vi "OnChunk.vi"(8 "Error In":errorcluster, 11 "JSON Tree In":variant) -> (0 "Error Out":errorcluster, 1 "Payload":variant, 2 "SessionId":string, 3 "JSON Tree Out":variant)   [LabVIEW 2017, in "LiteAgentSDK.lvlib"]
uses:
  LiteAgentSDK.lvlib
  <vilib>/LVH/i3 JSON/JSON Parsing/Get Object Parameter Files/Get Object Parameter - String.vi
  <vilib>/LVH/i3 JSON/JSON Parsing/Get Object Parameter Files/Get Object Parameter - Object.vi
  <vilib>/LVH/i3 JSON/i3-json.lvlib
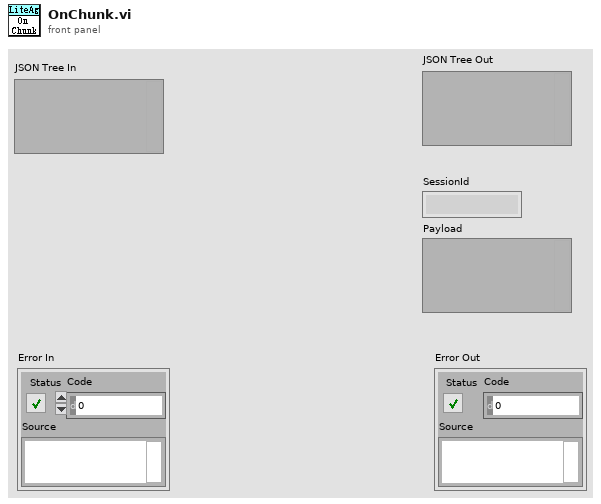
[diagram p1: front panel]
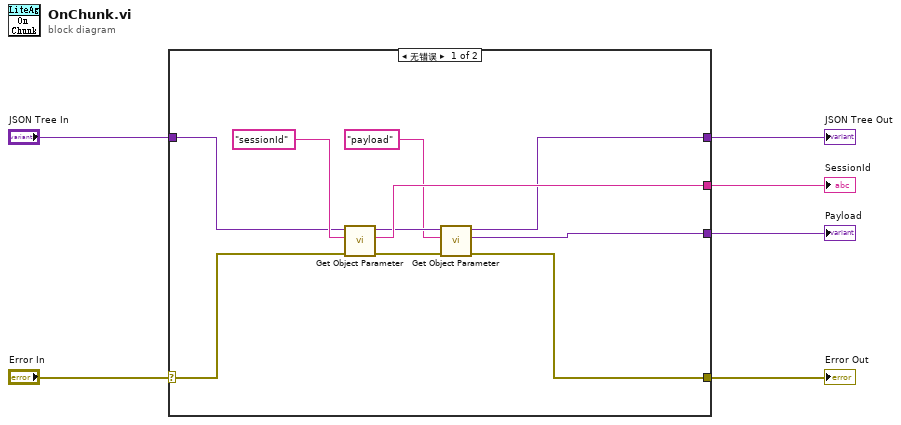
[diagram p0: block diagram]
diagram:
  n1 = case shown="无错误" "Error In" {
    selector: "Error In" -> [w13 w17]
    tunnel: [w11 w17] -> w5
    tunnel: "JSON Tree In" -> [w14 _]
    tunnel: [w15 _] -> w2
    tunnel: [w9 _] -> w3
    tunnel: [w7 _] -> w1
    frame No Error {
      n2 = call-poly <vilib>:"Get Object Parameter.vi"("error in (no error)"=w13, "Parameter Name"="sessionId", "JSON Tree In (JSON Object)"=w14) -> ("error out"=w12:errorcluster, "String Value"=w15:string, "JSON Tree Out Passthrough"=w10:variant)  [unwired: 5 in, 1 out]
      n3 = call-poly <vilib>:"Get Object Parameter.vi"("error in (no error)"=w12, "Parameter Name"="payload", "JSON Tree In (JSON Object)"=w10) -> ("error out"=w11:errorcluster, "JSON Object"=w7:variant, "JSON Tree Out Passthrough"=w9:variant)  [unwired: 5 in, 1 out]
    }
    frame Error {
    }
  }
  "Error Out" <- w5
  "JSON Tree Out" <- w3
  "SessionId" <- w2
  "Payload" <- w1
